vi "LineScanRemoteControl_withRotator.vi"() -> ()   [LabVIEW 2022 SP3]
uses:
  Control_LineScanRemoteControl.ctl
  Control_LineScanCounterAE.ctl
  D:/Dropbox/Members/Bragg, Alyssa/PolarizerRotator Folder/Control polarizer 1.ctl
panel:
  out "Elliptec Position":i32
  out "Elliptec error":errorcluster
  in  "Elliptec Address":refnum<visa-resource-name>
  in  "Rotation step size":dbl
  out "Last point\nduration (s)":dbl=5.42
  out "Current point":i32=1562
  out "Current\nAccumulation":i32=1
  in  "Finish point":bool
  in  "Next point":bool
  out "Linescan active":bool=TRUE
  in  "Halt program":bool
  in  "Stop linescan":bool
  in  "Start linescan":bool=TRUE
  in  "Total # of Accumulations":i32=4
  in  "# of Rotations":i32=1600 min=1 max=1000
  # "Linescan remote control"
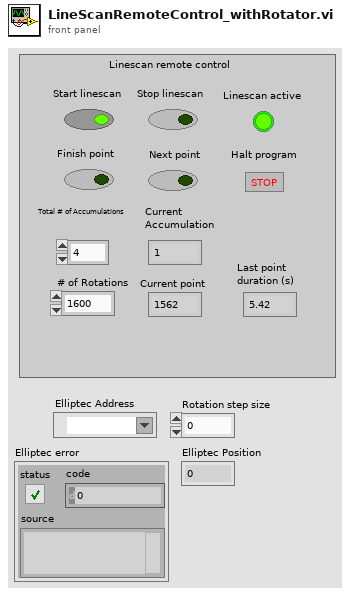
[diagram p1: front panel]
types:
  T1 = typedef "Control_LineScanRemoteControl.ctl" = enum16{"Start linescan", "Sit Idle", "Stop linescan", "Next Point", "Update from Counter", "Finish point", "Start DAQ control", "Poll DAQ control", "Stop DAQ control"}
  T2 = typedef "Control_LineScanCounterAE.ctl" = enum16{"Initialize", "Activate", "Attach indicators", "Increment Point", "Query", "Do Finish Point", "Acknowledge line", "Deactivate"}
  T3 = typedef "Control polarizer 1.ctl" = enum16{"Home", "Read position", "Go to position", "Jog", "Set jog size"}
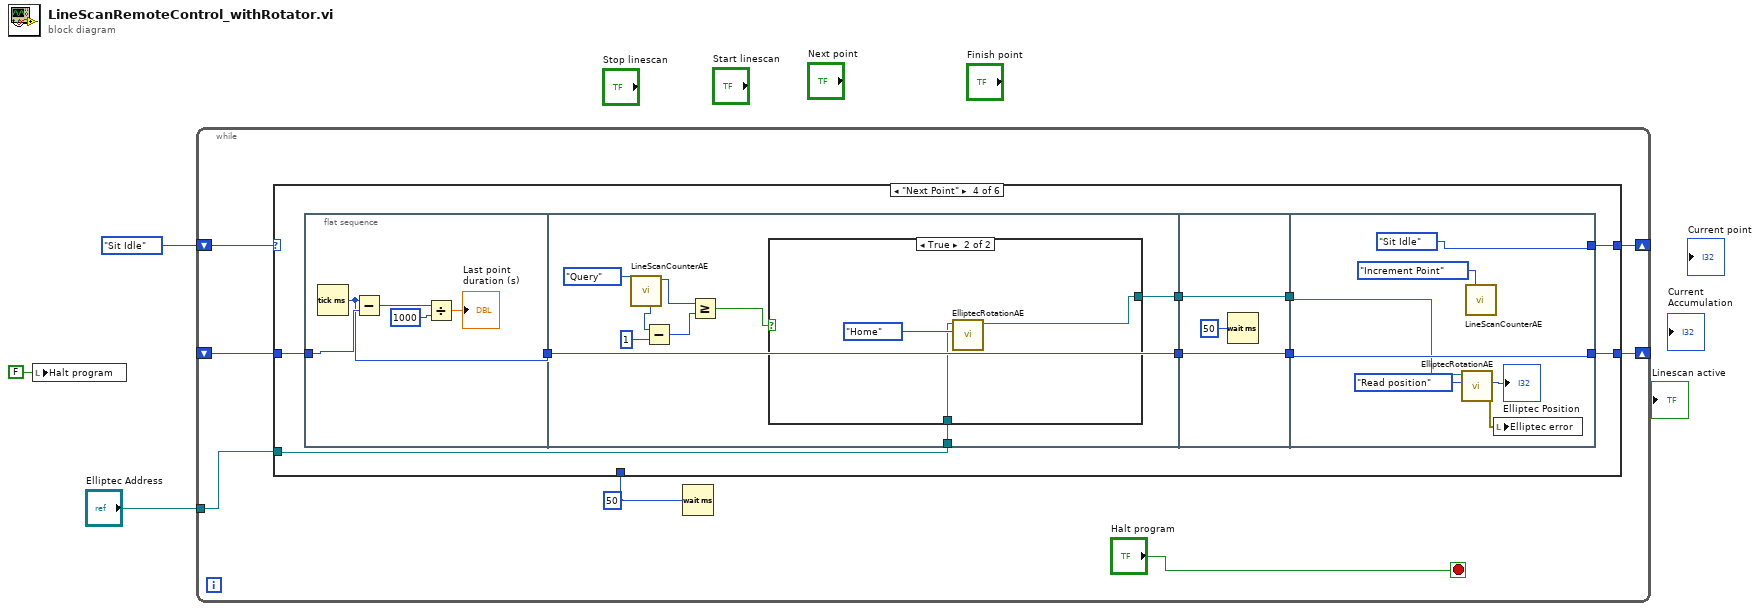
[diagram p0: block diagram]
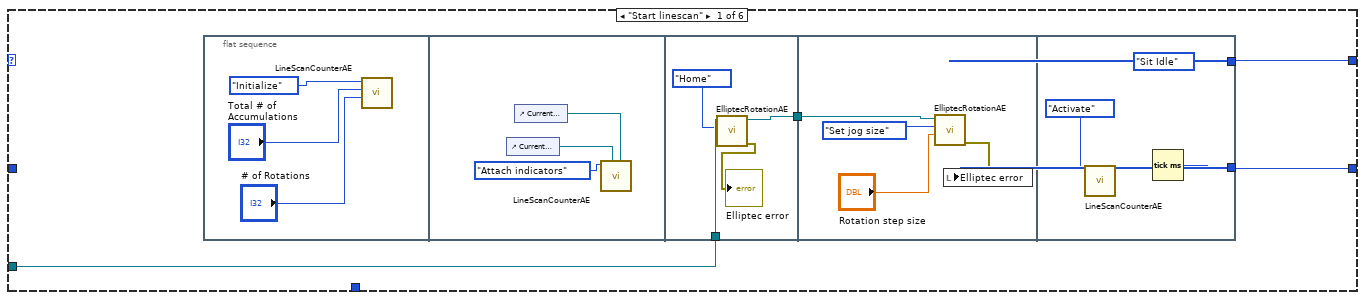
[diagram p2: hidden frame]
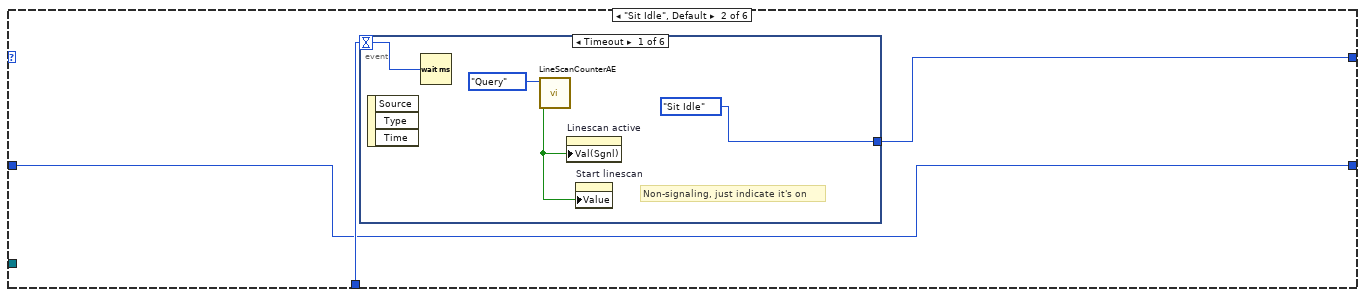
[diagram p3: hidden frame]
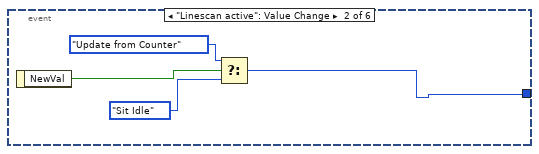
[diagram p4: hidden frame]
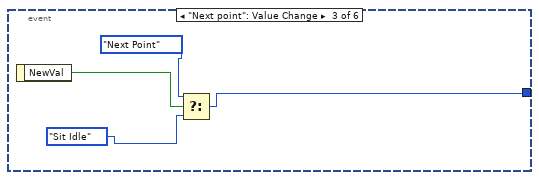
[diagram p5: hidden frame]
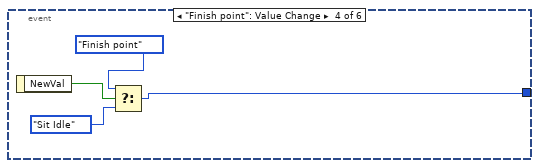
[diagram p6: hidden frame]
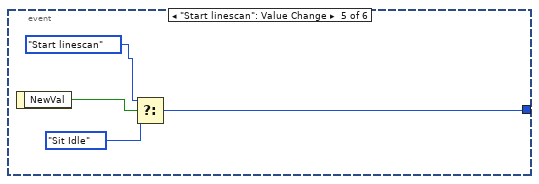
[diagram p7: hidden frame]
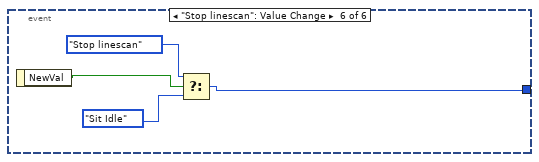
[diagram p8: hidden frame]
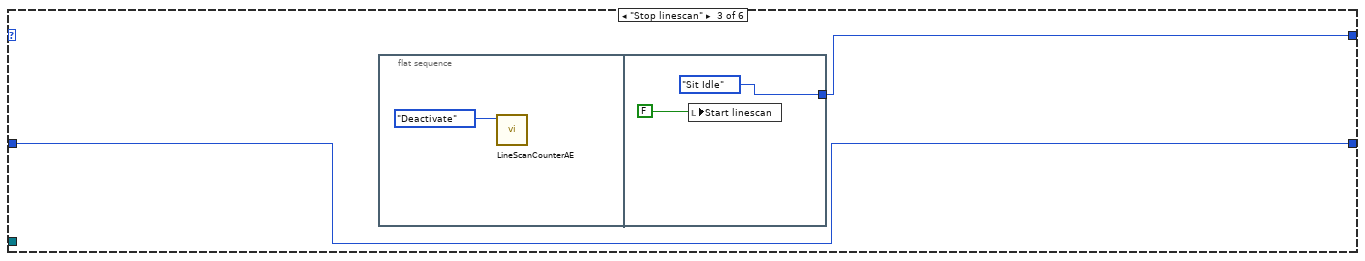
[diagram p9: hidden frame]
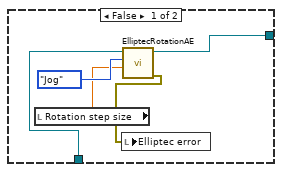
[diagram p10: hidden frame]
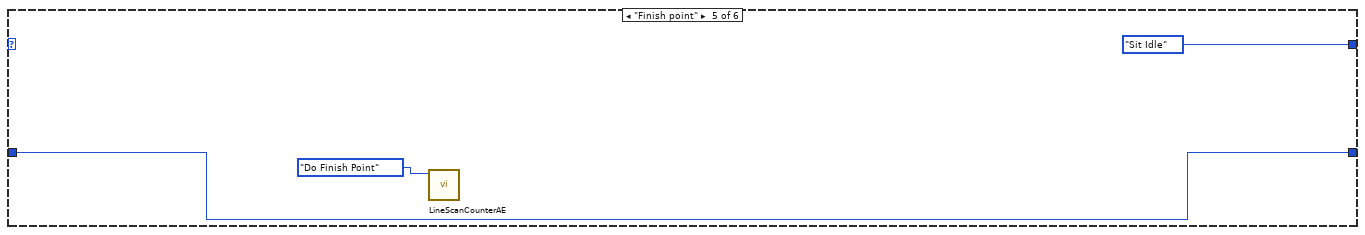
[diagram p11: hidden frame]
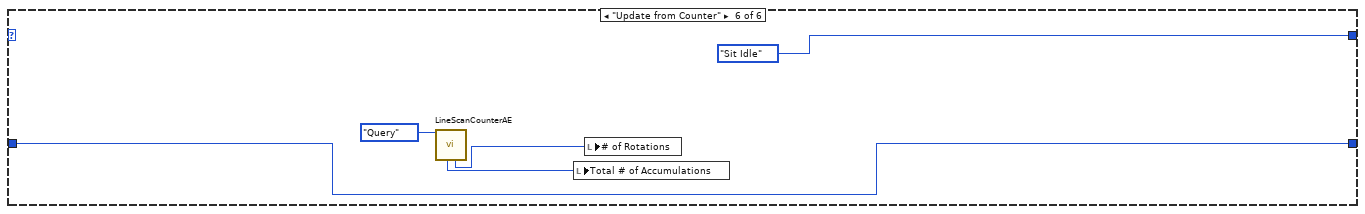
[diagram p12: hidden frame]
diagram:
  n1 = local write "Halt program"(FALSE ("Halt program")) -> ()
  n2 = while {
    shift-right: [w10] -> _
    shift-left: Control_LineScanRemoteControl."Sit Idle" -> [w7]
    shift-right: [w6] -> _
    shift-left: _ -> [w5]
    tunnel: "Elliptec Address" -> [w4]
    stop <- "Halt program" stop-if-true
    w8 = 50
    n3 = case shown="\"Next Point\"" w7 {
      tunnel: [w14 w33 w60 w69 Control_LineScanRemoteControl."Sit Idle" Control_LineScanRemoteControl."Sit Idle"] -> w10
      tunnel: w8 -> [_ w34 _ _ _ _]
      tunnel: [w13 w32 w59 w71 w106 w108] -> w6
      tunnel: w5 -> [_ w32 w59 w72 w106 w108]
      tunnel: w4 -> [w12 _ _ w68 _ _]
      frame "Start linescan" {
        n4 = flat-sequence {
          tunnel: w12 -> [w24]
          tunnel: [w23] -> w11
          tunnel: w11 -> [w25]
          tunnel: [Control_LineScanRemoteControl."Sit Idle"] -> w14
          tunnel: [w29] -> w13
          frame #0 {
            n5 = call "LineScanCounterAE.vi"("Number of points"="# of Rotations", "Accumulate to #"="Total # of Accumulations", "Task"=Control_LineScanCounterAE."Initialize" ("Enum")) -> ()  [unwired: 2 in, 7 out]
          }
          frame #1 {
            n6 = control-ref of="Current point"() -> (w20:refnum<vi>)
            n7 = control-ref of="Current\nAccumulation"() -> (w19:refnum<vi>)
            n8 = call "LineScanCounterAE.vi"("# Accumulated (reference)"=w19, "Current point index (reference)"=w20, "Task"=Control_LineScanCounterAE."Attach indicators" ("Enum")) -> ()  [unwired: 2 in, 7 out]
          }
          frame #2 {
            n9 = call "ElliptecRotationAE.vi"("Enum"=Control_polarizer_1."Home", "VISA Refnum in"=w24) -> ("error out"=→"Elliptec error":errorcluster, "VISA Refnum out"=w23:refnum<visa-resource-name>)  [unwired: 6 in, 2 out]
          }
          frame #3 {
            n10 = call "ElliptecRotationAE.vi"("Position or jog size"="Rotation step size", "Enum"=Control_polarizer_1."Set jog size", "VISA Refnum in"=w25) -> ("error out"=w26:errorcluster)  [unwired: 5 in, 3 out]
            n11 = local write "Elliptec error"(w26) -> ()
          }
          frame #4 {
            n12 = call "LineScanCounterAE.vi"("Task"=Control_LineScanCounterAE."Activate" ("Enum")) -> ()  [unwired: 4 in, 7 out]
            n13 = Tick Count (ms)() -> (millisecond timer value=w29:u32)
          }
        }
      }
      frame "Sit Idle", Default {
        n14 = event shown="[0] Timeout" {
          selector: _ -> [_ _ _ _ _ _]
          dyn-events: _ -> [_ _ _ _ _ _]
          timeout: w34 -> [w35 _ _ _ _ _]
          tunnel: [Control_LineScanRemoteControl."Sit Idle" w39 w45 w49 w53 w57] -> w33
          event Timeout {
            # "Non-signaling, just indicate it's on"
            n15 = event-data() -> ()  [unwired: 1 in, 3 out]
            n16 = Wait (ms)(milliseconds to wait=w35) -> ()  [unwired: 1 out]
            n17 = call "LineScanCounterAE.vi"("Task"=Control_LineScanCounterAE."Query" ("Enum")) -> ("Active"=w36:bool)  [unwired: 4 in, 6 out]
            n18 = property on="Linescan active" class="Bool (strict)"("Val(Sgnl)"=w36) -> ()  [unwired: 2 in, 2 out]
            n19 = property on="Start linescan" class="Bool (strict)"("Value"=w36) -> ()  [unwired: 2 in, 2 out]
          }
          event "Linescan active": Value Change {
            n20 = event-data() -> ("NewVal"=w40:bool)  [unwired: 1 in]
            n21 = Select(t=Control_LineScanRemoteControl."Update from Counter", s=w40, f=Control_LineScanRemoteControl."Sit Idle") -> (s? t:f=w39:T1)
          }
          event "Next point": Value Change {
            n22 = event-data() -> ("NewVal"=w46:bool)  [unwired: 1 in]
            n23 = Select(t=Control_LineScanRemoteControl."Next Point", s=w46, f=Control_LineScanRemoteControl."Sit Idle") -> (s? t:f=w45:T1)
          }
          event "Finish point": Value Change {
            n24 = event-data() -> ("NewVal"=w50:bool)  [unwired: 1 in]
            n25 = Select(t=Control_LineScanRemoteControl."Finish point", s=w50, f=Control_LineScanRemoteControl."Sit Idle") -> (s? t:f=w49:T1)
          }
          event "Start linescan": Value Change {
            n26 = event-data() -> ("NewVal"=w54:bool)  [unwired: 1 in]
            n27 = Select(t=Control_LineScanRemoteControl."Start linescan", s=w54, f=Control_LineScanRemoteControl."Sit Idle") -> (s? t:f=w53:T1)
          }
          event "Stop linescan": Value Change {
            n28 = event-data() -> ("NewVal"=w58:bool)  [unwired: 1 in]
            n29 = Select(t=Control_LineScanRemoteControl."Stop linescan", s=w58, f=Control_LineScanRemoteControl."Sit Idle") -> (s? t:f=w57:T1)
          }
        }
      }
      frame "Stop linescan" {
        n30 = flat-sequence {
          tunnel: [Control_LineScanRemoteControl."Sit Idle"] -> w60
          frame #0 {
            n31 = call "LineScanCounterAE.vi"("Task"=Control_LineScanCounterAE."Deactivate" ("Enum")) -> ()  [unwired: 4 in, 7 out]
          }
          frame #1 {
            n32 = local write "Start linescan"(FALSE ("Start linescan")) -> ()
          }
        }
      }
      frame "Next Point" {
        n33 = flat-sequence {
          tunnel: w72 -> [w77]
          tunnel: [w76] -> w70
          tunnel: w70 -> [w86]
          tunnel: [w86] -> w67
          tunnel: [w85] -> w65
          tunnel: w68 -> [w83]
          tunnel: w67 -> [w97]
          tunnel: [w97] -> w66
          tunnel: w65 -> [w96]
          tunnel: [w96] -> w64
          tunnel: w66 -> [w104]
          tunnel: w64 -> [w101]
          tunnel: [w104] -> w71
          tunnel: [Control_LineScanRemoteControl."Sit Idle"] -> w69
          frame #0 {
            n34 = Tick Count (ms)() -> (millisecond timer value=w76:u32)
            n35 = Subtract(x=w76, y=w77) -> (x-y=w75:u32)
            n36 = Divide(x=w75, y=1000) -> (x/y=→"Last point\nduration (s)":dbl)
          }
          frame #1 {
            n37 = call "LineScanCounterAE.vi"("Task"=Control_LineScanCounterAE."Query") -> ("Current point index"=w80:i32, "Number of points (query)"=w82:i32)  [unwired: 4 in, 5 out]
            n38 = Subtract(x=w82, y=1) -> (x-y=w79:i32)
            n39 = Greater Or Equal?(x=w80, y=w79) -> (x >= y?=w78:bool)
            n40 = case shown="True" w78 {
              tunnel: [w89 w92] -> w85
              tunnel: w83 -> [w87 w93]
              frame False {
                n41 = local read "Rotation step size"() -> (w88:dbl)
                n42 = call "ElliptecRotationAE.vi"("Position or jog size"=w88, "Enum"=Control_polarizer_1."Jog", "VISA Refnum in"=w87) -> ("error out"=w90:errorcluster, "VISA Refnum out"=w89:refnum<visa-resource-name>)  [unwired: 5 in, 2 out]
                n43 = local write "Elliptec error"(w90) -> ()
              }
              frame True {
                n44 = call "ElliptecRotationAE.vi"("Enum"=Control_polarizer_1."Home", "VISA Refnum in"=w93) -> ("VISA Refnum out"=w92:refnum<visa-resource-name>)  [unwired: 6 in, 3 out]
              }
            }
          }
          frame #2 {
            n45 = Wait (ms)(milliseconds to wait=u32 50) -> ()  [unwired: 1 out]
          }
          frame #3 {
            n46 = call "ElliptecRotationAE.vi"("Enum"=Control_polarizer_1."Read position", "VISA Refnum in"=w101) -> ("error out"=w98:errorcluster, "Read position"=→"Elliptec Position":i32)  [unwired: 6 in, 2 out]
            n47 = call "LineScanCounterAE.vi"("Task"=Control_LineScanCounterAE."Increment Point" ("Enum")) -> ()  [unwired: 4 in, 7 out]
            n48 = local write "Elliptec error"(w98) -> ()
          }
        }
      }
      frame "Finish point" {
        n49 = call "LineScanCounterAE.vi"("Task"=Control_LineScanCounterAE."Do Finish Point" ("Enum")) -> ()  [unwired: 4 in, 7 out]
      }
      frame "Update from Counter" {
        n50 = call "LineScanCounterAE.vi"("Task"=Control_LineScanCounterAE."Query" ("Enum")) -> ("Number of points (query)"=w112:i32, "Accumulate to (query)"=w111:i32)  [unwired: 4 in, 5 out]
        n51 = local write "Total # of Accumulations"(w111) -> ()
        n52 = local write "# of Rotations"(w112) -> ()
      }
    }
    n53 = Wait (ms)(milliseconds to wait=w8) -> ()  [unwired: 1 out]
  }
